vi "DefineNetCDFFile.vi"(0 "BaseFilePath":string="C:\\Users\\eol-lidar\\Desktop\\NetCDFTesting\\", 1 "InputFileName":string, 2 "AltitudeBins":dbl=560.0, 3 "WVDialNumber":dbl=2.0, 5 "ErrorIn":errorcluster) -> (14 "FullFileName":string="C:\\Users\\eol-lidar\\Desktop\\NetCDFTesting\\TestingNCARWVDIAL002_20171024_094408.cdf", 15 "BaseName":string, 19 "ErrorOut":errorcluster)   [LabVIEW 2012]
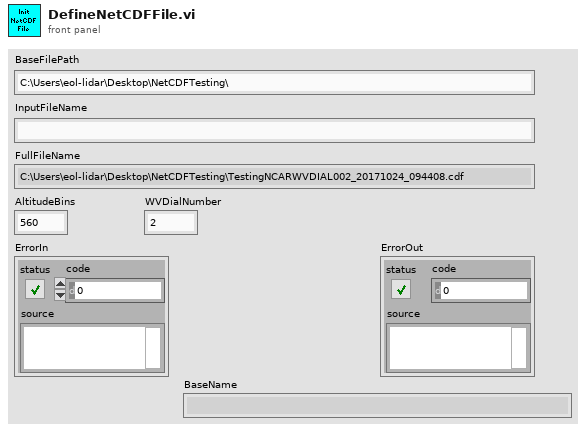
[diagram p1: front panel]
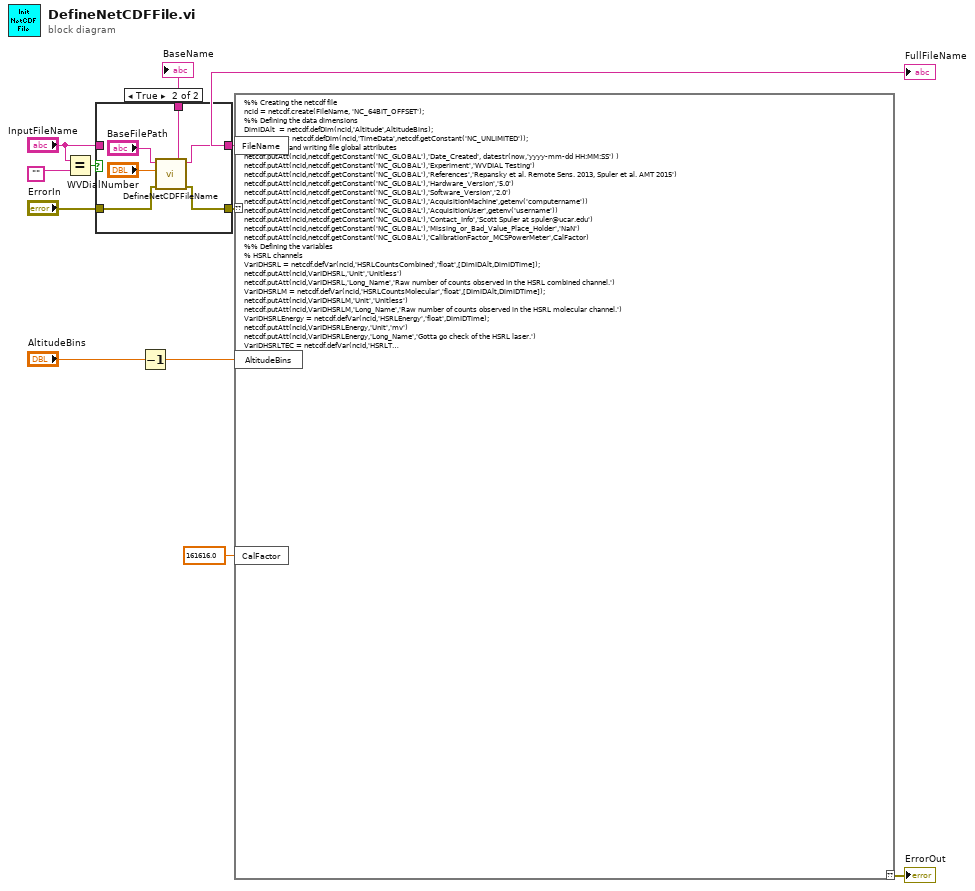
[diagram p0: block diagram]
diagram:
  n1 = Equal?(x="InputFileName", y="") -> (x = y?=w11:bool)
  n2 = case shown="True" w11 {
    tunnel: "InputFileName" -> [w12 _]
    tunnel: [w12 w19] -> w8
    tunnel: "ErrorIn" -> [w13 w18]
    tunnel: [w13 w17] -> w6
    tunnel: [w12 w14] -> w2
    frame False {
    }
    frame True {
      n3 = call "DefineNetCDFFileName.vi"("ErrorIn"=w18, "WVDialNumber"="WVDialNumber", "BasePath"="BaseFilePath") -> ("ErrorOut"=w17:errorcluster, "BaseName"=w14:string, "FullFileName"=w19:string)  [unwired: 6 in]
    }
  }
  "FullFileName" <- w8
  "BaseName" <- w2
  n4 = Decrement(x="AltitudeBins") -> (x-1=w3:dbl)
  n5 = script code="%% Creating the netcdf file\nncid = netcdf.create(FileName, 'NC_64BIT_OFFSET');\n%% Defining the data dimensions\nDimIDAlt  = netcdf.defDim(ncid,'Altitude',AltitudeBins);\nDimIDTime = netcdf.defDim(ncid,'TimeData',netcdf.getConstant('NC_UNLIMITED'));\n%% Defining and writing file global attributes \nnetcdf.putAtt(ncid,netcdf.getConstant('NC_GLOBAL'),'Date_Created', datestr(now,'yyyy-mm-dd HH:MM:SS') ) \nnetcdf.putAtt(ncid,netcdf.getConstant('NC_GLOBAL'),'Experiment','WVDIAL Testing') \nnetcdf.putAtt(ncid,netcdf.getConstant('NC_GLOBAL'),'References','Repansky et al. Remote Sens. 2013, Spuler et al. AMT 2015') \nnetcdf.putAtt(ncid,netcdf.getConstant('NC_GLOBAL'),'Hardware_Version','5.0')\nnetcdf.putAtt(ncid,netcdf.getConstant('NC_GLOBAL'),'Software_Version','2.0') \nnetcdf.putAtt(ncid,netcdf.getConstant('NC_GLOBAL'),'AcquisitionMachine',getenv('computername'))\nnetcdf.putAtt(ncid,netcdf.getConstant('NC_GLOBAL'),'AcquisitionUser',getenv('username'))\nnetcdf.putAtt(ncid,netcdf.getConstant('NC_GLOBAL'),'Contact_Info','Scott Spuler at spuler@ucar.edu') \nnetcdf.putAtt(ncid,netcdf.getConstant('NC_GLOBAL'),'Missing_or_Bad_Value_Place_Holder','NaN')\nnetcdf.putAtt(ncid,netcdf.getConstant('NC_GLOBAL'),'CalibrationFactor_MCSPowerMeter',CalFactor)\n%% Defining the variables\n% HSRL channels\nVarIDHSRL = netcdf.defVar(ncid,'HSRLCountsCombined','float',[DimIDAlt,DimIDTime]);\nnetcdf.putAtt(ncid,VarIDHSRL,'Unit','Unitless')\nnetcdf.putAtt(ncid,VarIDHSRL,'Long_Name','Raw number of counts observed in the HSRL combined channel.')\nVarIDHSRLM = netcdf.defVar(ncid,'HSRLCountsMolecular','float',[DimIDAlt,DimIDTime]);\nnetcdf.putAtt(ncid,VarIDHSRLM,'Unit','Unitless')\nnetcdf.putAtt(ncid,VarIDHSRLM,'Long_Name','Raw number of counts observed in the HSRL molecular channel.')\nVarIDHSRLEnergy = netcdf.defVar(ncid,'HSRLEnergy','float',DimIDTime);\nnetcdf.putAtt(ncid,VarIDHSRLEnergy,'Unit','mv')\nnetcdf.putAtt(ncid,VarIDHSRLEnergy,'Long_Name','Gotta go check of the HSRL laser.')\nVarIDHSRLTEC = netcdf.defVar(ncid,'HSRLTEC','float',DimIDTime);\nnetcdf.putAtt(ncid,VarIDHSRLTEC,'Unit','C')\nnetcdf.putAtt(ncid,VarIDHSRLTEC,'Long_Name','Thermo-electric cooler temperature of the HSRL laser.')\nVarIDHSRLLam = netcdf.defVar(ncid,'HSRLWavelength','float',DimIDTime);\nnetcdf.putAtt(ncid,VarIDHSRLLam,'Unit','nm')\nnetcdf.putAtt(ncid,VarIDHSRLLam,'Long_Name','Wavelength of the HSRL laser transmitter.')\n% Water vapor offline\nVarIDOffline = netcdf.defVar(ncid,'H2OOfflineCounts','float',[DimIDAlt,DimIDTime]);\nnetcdf.putAtt(ncid,VarIDOffline,'Unit','Unitless')\nnetcdf.putAtt(ncid,VarIDOffline,'Long_Name','Raw number of counts observed in the water vapor offline channel.')\nVarIDOfflineEnergy = netcdf.defVar(ncid,'H2OOfflineEnergy','float',DimIDTime);\nnetcdf.putAtt(ncid,VarIDOfflineEnergy,'Unit','mv')\nnetcdf.putAtt(ncid,VarIDOfflineEnergy,'Long_Name','Gotta go check of the water vapor offline laser.')\nVarIDOfflineTEC = netcdf.defVar(ncid,'H2OOfflineTEC','float',DimIDTime);\nnetcdf.putAtt(ncid,VarIDOfflineTEC,'Unit','C')\nnetcdf.putAtt(ncid,VarIDOfflineTEC,'Long_Name','Thermo-electric cooler temperature of the water vapor offline laser.')\nVarIDOfflineLam = netcdf.defVar(ncid,'H2OOfflineWavelength','float',DimIDTime);\nnetcdf.putAtt(ncid,VarIDOfflineLam,'Unit','nm')\nnetcdf.putAtt(ncid,VarIDOfflineLam,'Long_Name','Wavelength of the water vapor offline laser transmitter.')\n% Water vapor online \nVarIDOnline = netcdf.defVar(ncid,'H2OOnlineCounts','float',[DimIDAlt,DimIDTime]);\nnetcdf.putAtt(ncid,VarIDOnline,'Unit','Unitless')\nnetcdf.putAtt(ncid,VarIDOnline,'Long_Name','Raw number of counts observed in the water vapor online channel.')\nVarIDOnlineEnergy = netcdf.defVar(ncid,'H2OOnlineEnergy','float',DimIDTime);\nnetcdf.putAtt(ncid,VarIDOnlineEnergy,'Unit','mv')\nnetcdf.putAtt(ncid,VarIDOnlineEnergy,'Long_Name','Gotta go check of the online laser.')\nVarIDOnlineTEC = netcdf.defVar(ncid,'H2OOnlineTEC','float',DimIDTime);\nnetcdf.putAtt(ncid,VarIDOnlineTEC,'Unit','C')\nnetcdf.putAtt(ncid,VarIDOnlineTEC,'Long_Name','Thermo-electric cooler temperature of the online laser.')\nVarIDOnlineLam = netcdf.defVar(ncid,'H2OOnlineWavelength','float',DimIDTime);\nnetcdf.putAtt(ncid,VarIDOnlineLam,'Unit','nm')\nnetcdf.putAtt(ncid,VarIDOnlineLam,'Long_Name','Wavelength of the water vapor online laser transmitter.')\n% Meta data\nVarIDAccu = netcdf.defVar(ncid,'NumberOfAccumulations','float',DimIDTime);\nnetcdf.putAtt(ncid,VarIDAccu,'Unit','Unitless')\nnetcdf.putAtt(ncid,VarIDAccu,'Long_Name','Number of laser shots per profile of data taken.')\nVarIDEtWV = netcdf.defVar(ncid,'ReceiverEtalonTempWV','float',DimIDTime);\nnetcdf.putAtt(ncid,VarIDEtWV,'Unit','C')\nnetcdf.putAtt(ncid,VarIDEtWV,'Long_Name','Water vapor receiver etalon temperature.')\nVarIDEtHSRL = netcdf.defVar(ncid,'ReceiverEtalonTempHSRL','float',DimIDTime);\nnetcdf.putAtt(ncid,VarIDEtHSRL,'Unit','C')\nnetcdf.putAtt(ncid,VarIDEtHSRL,'Long_Name','HSRL receiver etalon temperature.')\nVarIDTimePB = netcdf.defVar(ncid,'TimePerBin','float',DimIDTime);\nnetcdf.putAtt(ncid,VarIDTimePB,'Unit','ns')\nnetcdf.putAtt(ncid,VarIDTimePB,'Long_Name','Time of flight of each multi-channel scaler data bin.')\nVarIDTime = netcdf.defVar(ncid,'Time','float',DimIDTime);\nnetcdf.putAtt(ncid,VarIDTime,'Unit','UTC')\nnetcdf.putAtt(ncid,VarIDTime,'Long_Name','Fractional day of year of the data time.eg: 2.5 is Noon on January, 2nd.')\n% Weather station\nVarIDWSAH = netcdf.defVar(ncid,'WSAbsoluteHumidity','float',DimIDTime);\nnetcdf.putAtt(ncid,VarIDWSAH,'Unit','g/kg')\nnetcdf.putAtt(ncid,VarIDWSAH,'Long_Name','Absolute humidity read by the weather station.')\nVarIDWSP = netcdf.defVar(ncid,'WSPressure','float',DimIDTime);\nnetcdf.putAtt(ncid,VarIDWSP,'Unit','mb')\nnetcdf.putAtt(ncid,VarIDWSP,'Long_Name','Pressure read by the weather station.')\nVarIDWSRH = netcdf.defVar(ncid,'WSRelativeHumidity','float',DimIDTime);\nnetcdf.putAtt(ncid,VarIDWSRH,'Unit','%')\nnetcdf.putAtt(ncid,VarIDWSRH,'Long_Name','Relative humidity read by the weather station.')\nVarIDWST = netcdf.defVar(ncid,'WSTemperature','float',DimIDTime);\nnetcdf.putAtt(ncid,VarIDWST,'Unit','C')\nnetcdf.putAtt(ncid,VarIDWST,'Long_Name','Temperature read by the weather station.')\n%% CLosing the netcdf file\nnetcdf.close(ncid)" ("Script Node")("??"=w6, "FileName"=w8, "AltitudeBins"=w3, "CalFactor"=161616.0 ("Real")) -> ("??"=→"ErrorOut":errorcluster)
